vi "JSON Add White Space.vi"(8 "error in (no error)":errorcluster, 11 "JSON string":string) -> (0 "error out":errorcluster, 3 "Modified JSON string":string)   [LabVIEW 2020, in "File IO.lvlib" / "JSON Utilities.lvlib"]
doc: "Adds white space to a string generated by the Flatten to JSON String VI."
uses:
  JSON Utilities.lvlib
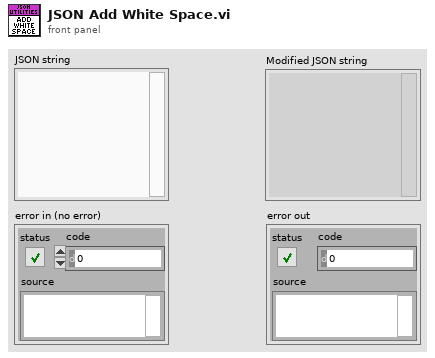
[diagram p1: front panel]
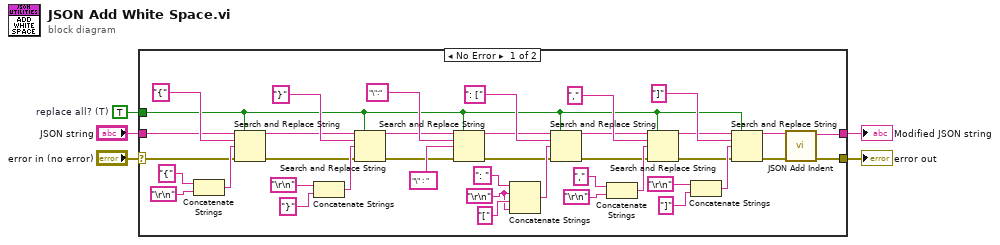
[diagram p0: block diagram]
diagram:
  w1 = TRUE  # replace all? (T)
  n1 = case shown="No Error" "error in (no error)" {
    selector: "error in (no error)" -> [w10 w46]
    tunnel: "JSON string" -> [w12 w47]
    tunnel: [w6 w47] -> w4
    tunnel: [w8 w46] -> w3
    tunnel: w1 -> [w9 _]
    frame No Error {
      w13 = "\r\n"
      n2 = Concatenate Strings("{" ("replace string (\"\")"), "\r\n") -> (w42:string)
      n3 = Search and Replace String(replace all?=w9, input string=w12, search string="{", replace string=w42, error in=w10) -> (result string=w38:string, error out=w39:errorcluster)  [unwired: 3 in, 2 out]
      n4 = Concatenate Strings("\r\n", "}" ("replace string (\"\")")) -> (w40:string)
      n5 = Search and Replace String(replace all?=w9, input string=w38, search string="}", replace string=w40, error in=w39) -> (result string=w33:string, error out=w32:errorcluster)  [unwired: 3 in, 2 out]
      n6 = Search and Replace String(replace all?=w9, input string=w33, search string="\":", replace string="\" : " ("replace string (\"\")"), error in=w32) -> (result string=w27:string, error out=w28:errorcluster)  [unwired: 3 in, 2 out]
      n7 = Concatenate Strings(": " ("replace string (\"\")"), w13, "[" ("string"), w13) -> (w29:string)
      n8 = Search and Replace String(replace all?=w9, input string=w27, search string=": [", replace string=w29, error in=w28) -> (result string=w22:string, error out=w21:errorcluster)  [unwired: 3 in, 2 out]
      n9 = Concatenate Strings("," ("replace string (\"\")"), "\r\n") -> (w23:string)
      n10 = Search and Replace String(replace all?=w9, input string=w22, search string=",", replace string=w23, error in=w21) -> (result string=w16:string, error out=w15:errorcluster)  [unwired: 3 in, 2 out]
      n11 = Concatenate Strings("\r\n", "]" ("replace string (\"\")")) -> (w19:string)
      n12 = Search and Replace String(replace all?=w9, input string=w16, search string="]", replace string=w19, error in=w15) -> (result string=w7:string, error out=w11:errorcluster)  [unwired: 3 in, 2 out]
      n13 = call "JSON Add Indent.vi"("error in (no error)"=w11, "JSON String"=w7) -> ("error out"=w8:errorcluster, "Indented JSON String"=w6:string)  [unwired: 8 in]
    }
    frame Error {
    }
  }
  "Modified JSON string" <- w4
  "error out" <- w3
